vi "toJSON.vi"(8 "error in (no error)":errorcluster, 11 "tBSONDocument in":refnum<class "tBSONDocument.lvclass">) -> (0 "error out":errorcluster, 2 "JSON":string, 3 "tBSONDocument out":refnum<class "tBSONDocument.lvclass">)   [LabVIEW 2013, in "BSON.lvlib" / "tBSONDocument.lvclass"]
doc: "VI converts this document into a string containing a JSON object of its contents. This will recursively traverse documents contained inside this document."
uses:
  tBSONDocument.lvclass
  tBSONDocument.lvclass/tBSONDocument.ctl
  tBSONElement/tBSONElement.lvclass
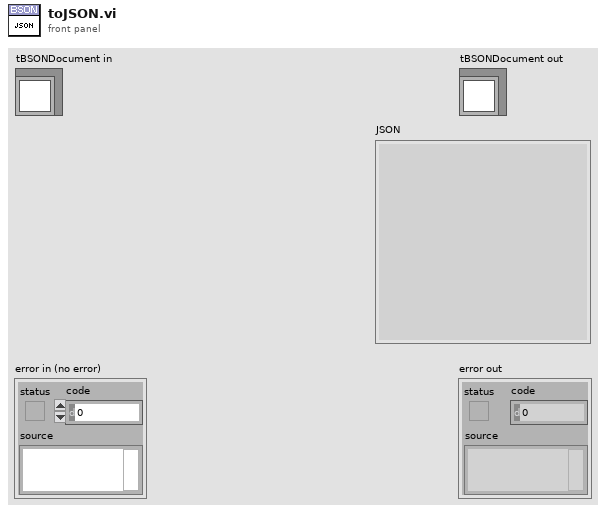
[diagram p1: front panel]
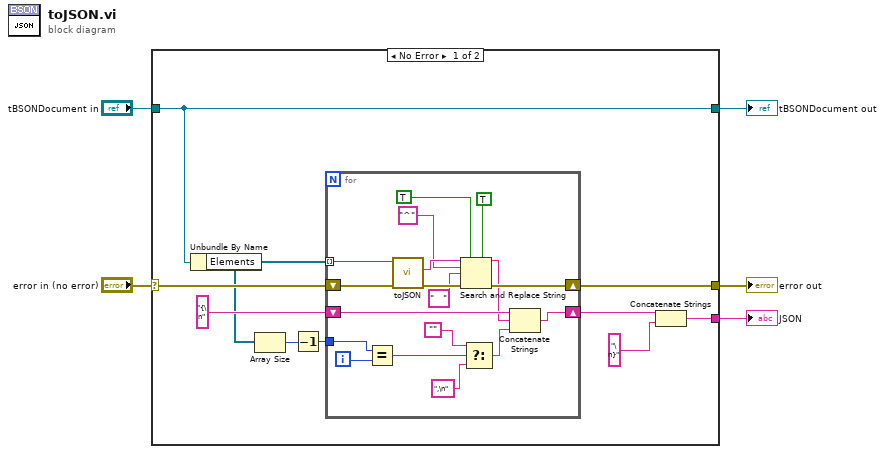
[diagram p0: block diagram]
diagram:
  n1 = case shown="No Error" "error in (no error)" {
    selector: "error in (no error)" -> [w14 w35]
    tunnel: [w9 w35] -> w4
    tunnel: [w13 w34] -> w2
    tunnel: "tBSONDocument in" -> [w13 w34]
    tunnel: [w10 _] -> w1
    frame No Error {
      n2 = Unbundle By Name(w13) -> ("Elements"=w7:refnum<class "tBSONElement.lvclass">[])
      n3 = Array Size(array=w7) -> (size(s)=w8:i32)
      n4 = Decrement(x=w8) -> (x-1=w6:i32)
      n5 = for {
        shift-right: [w31] -> w12
        shift-left: "{\n" -> [w30]
        shift-right: [w23] -> w9
        shift-left: w14 -> [w33]
        tunnel: w7 -> [w32] mode=indexing
        tunnel: w6 -> [w20]
        i -> [w21]
        n6 = Equal?(x=w20, y=w21) -> (x = y?=w17:bool)
        n7 = call-dynamic "toJSON.vi"("error in (no error)"=w33, "tBSONElement in"=w32) -> ("error out"=w29:errorcluster, "JSON"=w28:string)  [unwired: 7 in, 1 out]
        n8 = Search and Replace String(replace all?=TRUE ("replace all? (F)"), multiline?=TRUE ("multiline? (F)"), input string=w28, search string="^", replace string="   " ("replace string (\"\")"), error in=w29) -> (result string=w22:string, error out=w23:errorcluster)  [unwired: 2 in, 2 out]
        n9 = Select(t="", s=w17, f=",\n" ("string")) -> (s? t:f=w16:string)
        n10 = Concatenate Strings(w30, w22, w16) -> (w31:string)
      }
      n11 = Concatenate Strings(w12, "\n}") -> (w10:string)
    }
    frame Error {
    }
  }
  "error out" <- w4
  "tBSONDocument out" <- w2
  "JSON" <- w1
